vi "Calibrate Camera.vi"(0 "camID":i32, 1 "Board Type":T2, 2 "Board Size":T1={"Cols"=9, "Rows"=6}, 5 "error in (no error)":errorcluster, 6 "Zero Tangent Dist":bool, 7 "Skip Keys":bool, 8 "Aspect Ratio":bool=TRUE, 9 "Frames":i32=20, 10 "Fix Principal Point":bool=TRUE, 11 "Frameskip":i32=10) -> (14 "averageError":dbl, 15 "camMatrix":dbl[][](array[numeric]) caption="(fx, 0, cx;\n 0, fy, cy;\n 0, 0, 1)", 16 "distMatrix":dbl[](array[numeric]) caption="(k1, k2, p1, p2, k3)", 19 "error out":errorcluster)   [LabVIEW 2014, in "MSC Image.lvclass"]
doc: "Using this procedure you can calibrate your camera in terms of fish-eye effects and non-parrallelity of the camera sensor to the lens. A calibration board is needed for this.\nThe estimation of the camera matrix and distortion matrix is only required once for each fixed focus camera. \n\nFor more information about this process please check the documentation."
uses:
  MSC Image.lvclass
  controls/Camera Calibration Board Type.ctl
  controls/Size.ctl
  Dependencies/x86/MSC I Process32.dll
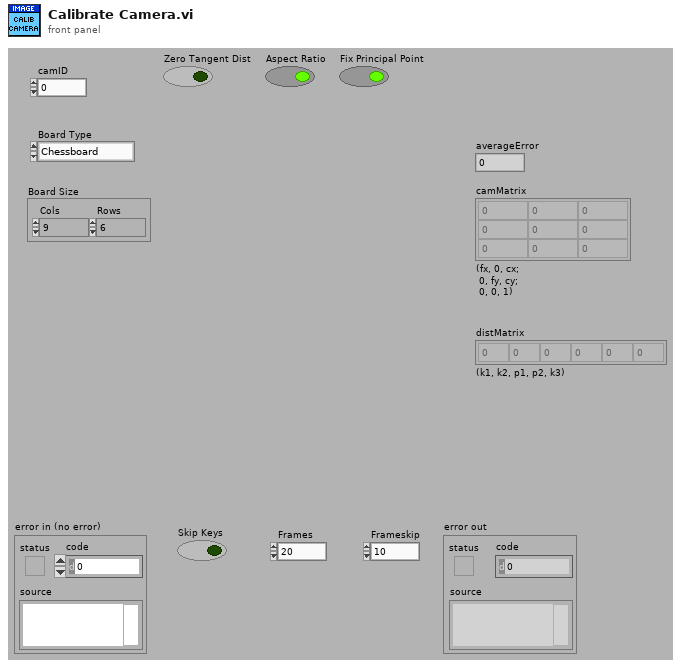
[diagram p1: front panel]
types:
  T1 = typedef "MSC Image.lvclass/Size.ctl" = cluster{"Cols":i32, "Rows":i32}
  T2 = typedef "MSC Image.lvclass/Camera Calibration Board Type.ctl" = enum16{"Chessboard", "Circles", "Asymmetric Circles"}
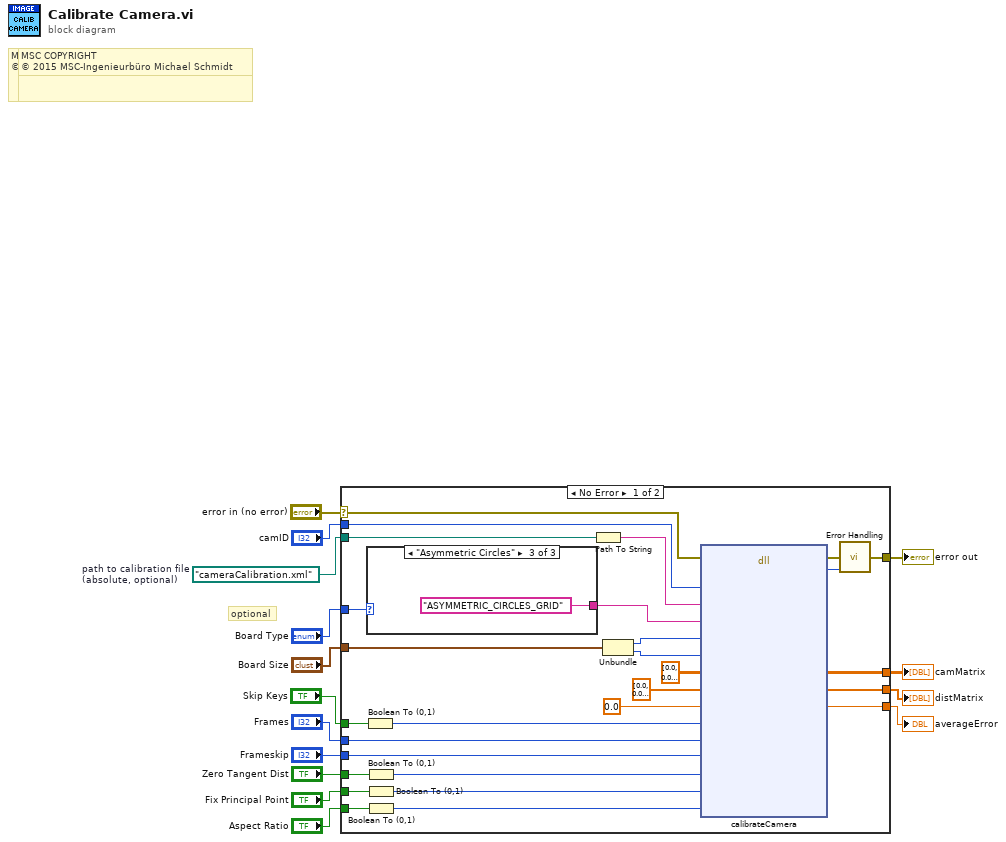
[diagram p0: block diagram]
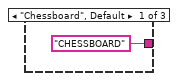
[diagram p2: hidden frame]
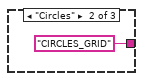
[diagram p3: hidden frame]
diagram:
  w14 = path "cameraCalibration.xml"  # path to calibration file (absolute, optional)
  # "MSC COPYRIGHT\n© 2016 MSC-Ingenieurbüro Michael Schmidt"
  # "MSC COPYRIGHT\n© 2016 MSC-Ingenieurbüro Michael Schmidt"
  # "MSC COPYRIGHT\n© 2015 MSC-Ingenieurbüro Michael Schmidt"
  # "MSC COPYRIGHT\n© 2015 MSC-Ingenieurbüro Michael Schmidt"
  # "optional"
  n1 = case shown="No Error" "error in (no error)" {
    selector: "error in (no error)" -> [w39 w47]
    tunnel: "camID" -> [w41 _]
    tunnel: [w40 w47] -> w1
    tunnel: w14 -> [w34 _]
    tunnel: "Board Type" -> [w33 _]
    tunnel: "Board Size" -> [w31 _]
    tunnel: "Frameskip" -> [w28 _]
    tunnel: "Frames" -> [w27 _]
    tunnel: "Zero Tangent Dist" -> [w26 _]
    tunnel: "Fix Principal Point" -> [w25 _]
    tunnel: "Aspect Ratio" -> [w24 _]
    tunnel: [w21 _] -> w6
    tunnel: [w20 _] -> w5
    tunnel: [w18 _] -> w4
    tunnel: "Skip Keys" -> [w16 _]
    frame No Error {
      n2 = Boolean To (0,1)(Boolean=w16) -> (0, 1=w17:i16)
      n3 = Boolean To (0,1)(Boolean=w26) -> (0, 1=w36:i16)
      n4 = Boolean To (0,1)(Boolean=w25) -> (0, 1=w38:i16)
      n5 = Boolean To (0,1)(Boolean=w24) -> (0, 1=w37:i16)
      n6 = case shown="\"Asymmetric Circles\"" w33 {
        tunnel: ["CHESSBOARD" ("boardType") "CIRCLES_GRID" ("boardType") "ASYMMETRIC_CIRCLES_GRID" ("boardType")] -> w32
        frame "Chessboard", Default {
        }
        frame "Circles" {
        }
        frame "Asymmetric Circles" {
        }
      }
      n7 = Path To String(path=w34) -> (string=w35:string)
      n8 = Unbundle(w31) -> ("Cols"=w30:i32, "Rows"=w29:i32)
      n9 = dll-call lib="C:/Users/MSC/LabVIEW Projekte/LV 2014/MSC I-Process/user.lib/MSC-I Process/Dependencies/x86/MSC I Process*.dll" fn="calibrateCamera"(error in=w39, "camID"=w41, "pathString"=w35, "boardType"=w32, "boardWidth"=w30, "boardHeight"=w29, "camMatrix"=dbl[][] [[0.0, 0.0, 0.0], [0.0, 0.0, 0.0], [0.0, 0.0, 0.0]] ("Camera matrix"), "distMatrix"=dbl[] [0.0, 0.0, 0.0, 0.0, 0.0] ("Distortion matrix"), "averageError"=0.0 ("reProjectionError"), "skipKeys"=w17, "frames"=w27, "frameskip"=w28, "calibZeroTangentDist"=w36, "calibFixPrincipalPoint"=w38, "aspectRatio"=w37) -> (error out=w42:errorcluster, "error"=w43:i32, "camMatrix"=w21:dbl[][], "distMatrix"=w20:dbl[], "averageError"=w18:dbl)  [unwired: 13 in, 1 out]
      n10 = call "Error Handling.vi"("error in (no error)"=w42, "return type"=w43) -> ("error out"=w40:errorcluster)  [unwired: 12 in, 1 out]
    }
    frame Error {
    }
  }
  "error out" <- w1
  "distMatrix" <- w5
  "camMatrix" <- w6
  "averageError" <- w4
